vi "ExSubWaitSpec.vi"(2 "error in (no error)":errorcluster, 3 "Spectrometer Handle":u32) -> (0 "error out":errorcluster, 1 "Spectrometer handle":u32)   [LabVIEW 2018]
panel:
  # "ExSubWaitSpec:\nThis Sub-VI waits for a spectograph\noperation to complete."
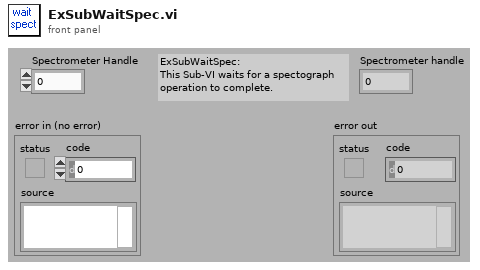
[diagram p1: front panel]
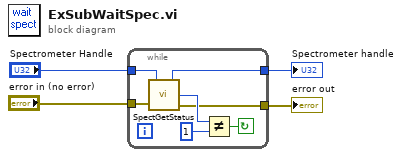
[diagram p0: block diagram]
diagram:
  n1 = while {
    tunnel: "Spectrometer Handle" -> [w8]
    tunnel: "error in (no error)" -> [w7]
    tunnel: [w6] -> w1
    tunnel: [w5] -> w2
    stop <- w9 continue-if-true
    n2 = call "SpectGetStatus.vi"("Spectrometer Handle"=w8, "error in"=w7) -> ("Spectrometer Handle"=w6:u32, "Command Status"=w10:u32, "error out"=w5:errorcluster)
    n3 = Not Equal?(x=w10, y=u32 1) -> (x != y?=w9:bool)
  }
  "error out" <- w2
  "Spectrometer handle" <- w1
